vi "Open_Mercury_connection.vi"(3 "IP Address":string="172.25.187.204") -> (0 "error out":errorcluster, 1 "Mercury Reference Out":T1)   [LabVIEW 2016]
uses:
  Equipment/Mercury iXX/Public/Controls/Mercury Reference.ctl
  Equipment/Mercury iXX/Public/Controls/Comms Transport Layer.ctl
  Equipment/Mercury iXX/Private/Controls/Query Dynamic Reference.ctl
  Equipment/Mercury iXX/Public/Controls/Serial Settings.ctl
  Equipment/Mercury iXX/Public/Libraries/System/Open/Open System.vi
  Equipment/Mercury iXX/Mercury iXX.lvlib
  Equipment/Mercury iXX/Public/Libraries/System.lvlib
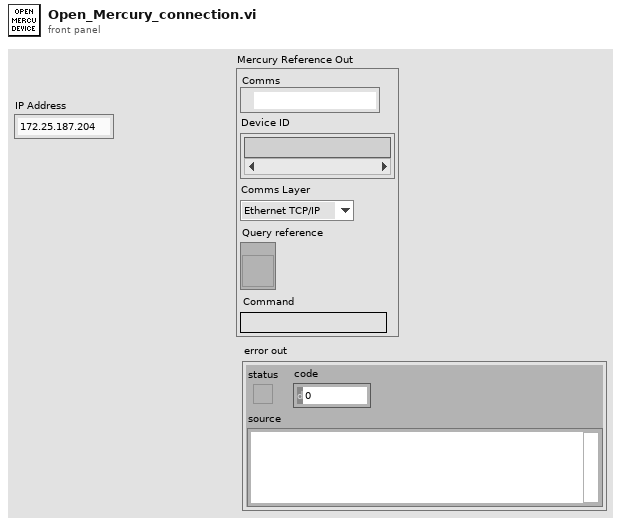
[diagram p1: front panel]
types:
  T1 = typedef "Mercury iXX.lvlib/Mercury Reference.ctl" = cluster{"Comms":refnum<visa-resource-name>, "Device ID":string[], "Comms Layer":T2, "Command":string, "Query reference":T3}
  T2 = typedef "Mercury iXX.lvlib/Comms Transport Layer.ctl" = enum16{"Ethernet TCP/IP", "USB", "ISOBus - RS-232", "GPIB"}
  T3 = typedef "Mercury iXX.lvlib/Query Dynamic Reference.ctl" = refnum<vi>
  T4 = typedef "Mercury iXX.lvlib/Serial Settings.ctl" = cluster{"Baud Rate":u32, "Parity":u16, "Data Bits":u16, "Stop Bits":u16, "Flow Control":u16}
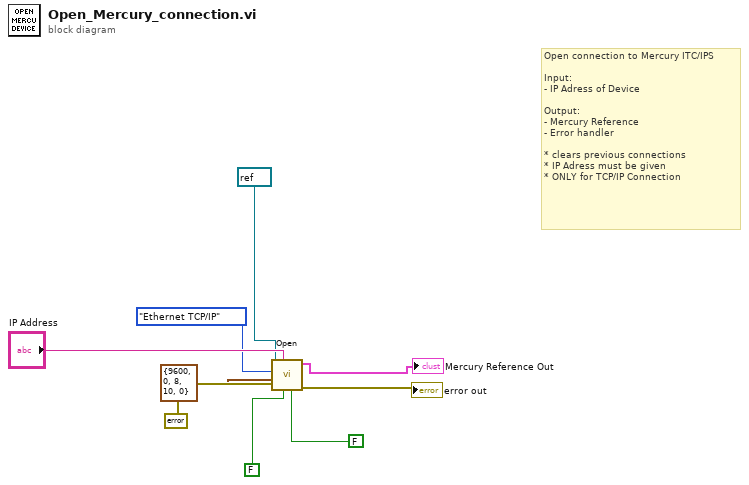
[diagram p0: block diagram]
diagram:
  # "Open connection to Mercury ITC/IPS\n\nInput:\n- IP Adress of Device\n\nOutput:\n- Mercury Reference\n- Error handler\n\n* clears previous connections\n* IP Adress must be given\n* ONLY for TCP/IP Connection"
  n1 = call-poly "Open.vi"("Clear Previous Connections (False)"=FALSE, "ID Query (True)"=FALSE, "IP Address"="IP Address", "error in (no error)"=errorcluster {"status"=FALSE, "code"=0, "source"=""}, "Serial Configuration"=T4 {"Baud Rate"=9600, "Parity"=0, "Data Bits"=8, "Stop Bits"=10, "Flow Control"=0}, "Comms Layer"=Comms_Transport_Layer."Ethernet TCP/IP", "VISA resource name"=refnum<visa-resource-name> refnum) -> ("error out"=→"error out":errorcluster, "Mercury Reference Out"=→"Mercury Reference Out":T1)  [unwired: 3 out]
